vi "8-bit video export-generate images.vi"(0 "AVI2 split file ref":T3, 1 "rgb Image":T2, 2 "Caller (exporter)":enum16{"Viewer", "Exporter"}(ring)=enum."Exporter", 3 "Initial frame":bool, 5 "Gobal frame number in time series data /master video (1 based)":i32, 7 "Split time series file frame index (0 based)":u32, 9 "I16 Image ref in":T2, 11 "Ctrl refs":T1, 12 "U8 Image ref in":T2, 13 "Whole dataset":bool) -> (4 "U8 Image":T2, 6 "Max intensity value":dbl, 10 "I16 Image":T2, 15 "error out":errorcluster)   [LabVIEW 2020]
uses:
  <vilib>/vision/Avi.llb/IMAQ AVI2 Refnum.ctl
  <vilib>/vision/Image Controls.llb/IMAQ Image.ctl
  Typedefs/8-bit video export window ctrl refs.ctl
  Patch-Vol video generator/Typedefs/Bright-Contr-Gamma cluster.ctl
  Typedefs/Speed graph behaviour enum.ctl
panel:
  in  "Output X Resolution per Tier":i32=500
  out "Image Pixels (U32)":u32[][](array[numeric])
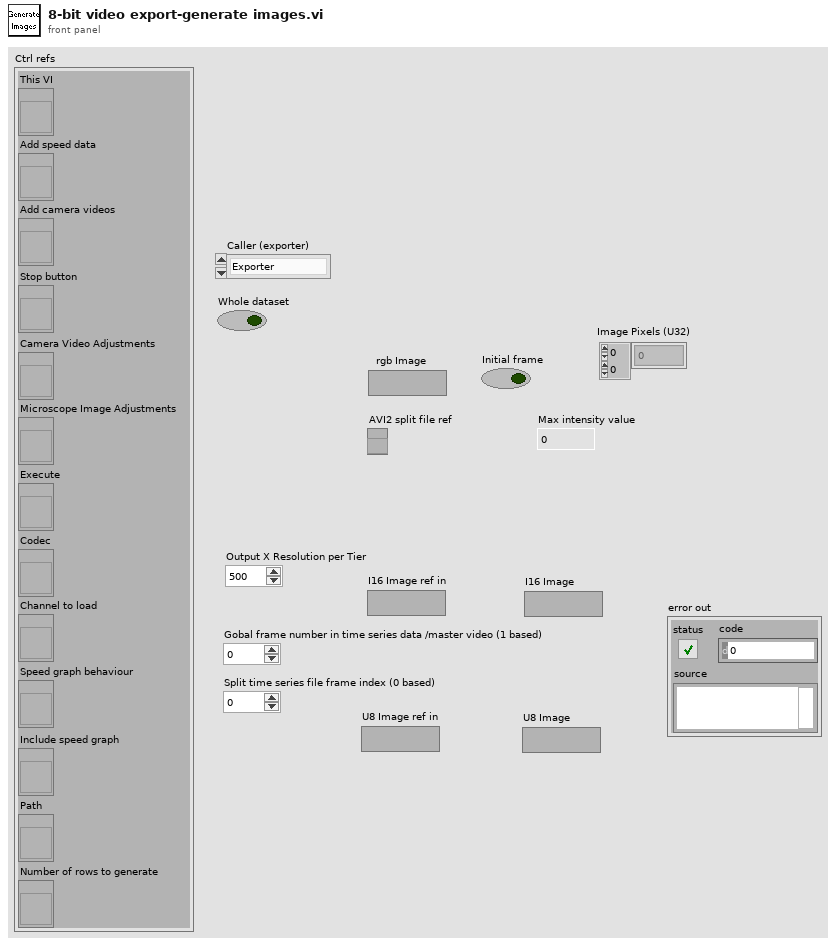
[diagram p1: front panel]
types:
  T1 = typedef "8-bit video export window ctrl refs.ctl" = cluster{"This VI":refnum<vi>, "Add speed data":refnum<vi>, "Add camera videos":refnum<vi>, "Stop button":refnum<vi>, "Camera Video Adjustments":refnum<vi>, "Microscope Image Adjustments":refnum<vi>, "Execute":refnum<vi>, "Codec":refnum<vi>, "Channel to load":refnum<vi>, "Speed graph behaviour":refnum<vi>, "Include speed graph":refnum<vi>, "Number of rows to generate":refnum<vi>, "Path":refnum<vi>}
  T2 = typedef "IMAQ Image.ctl" = refnum<image>
  T3 = typedef "IMAQ AVI2 Refnum.ctl" = refnum<k20>
  T4 = typedef "Bright-Contr-Gamma cluster.ctl" = cluster{"Brightness":sgl, "Contrast":sgl, "Gamma":sgl}
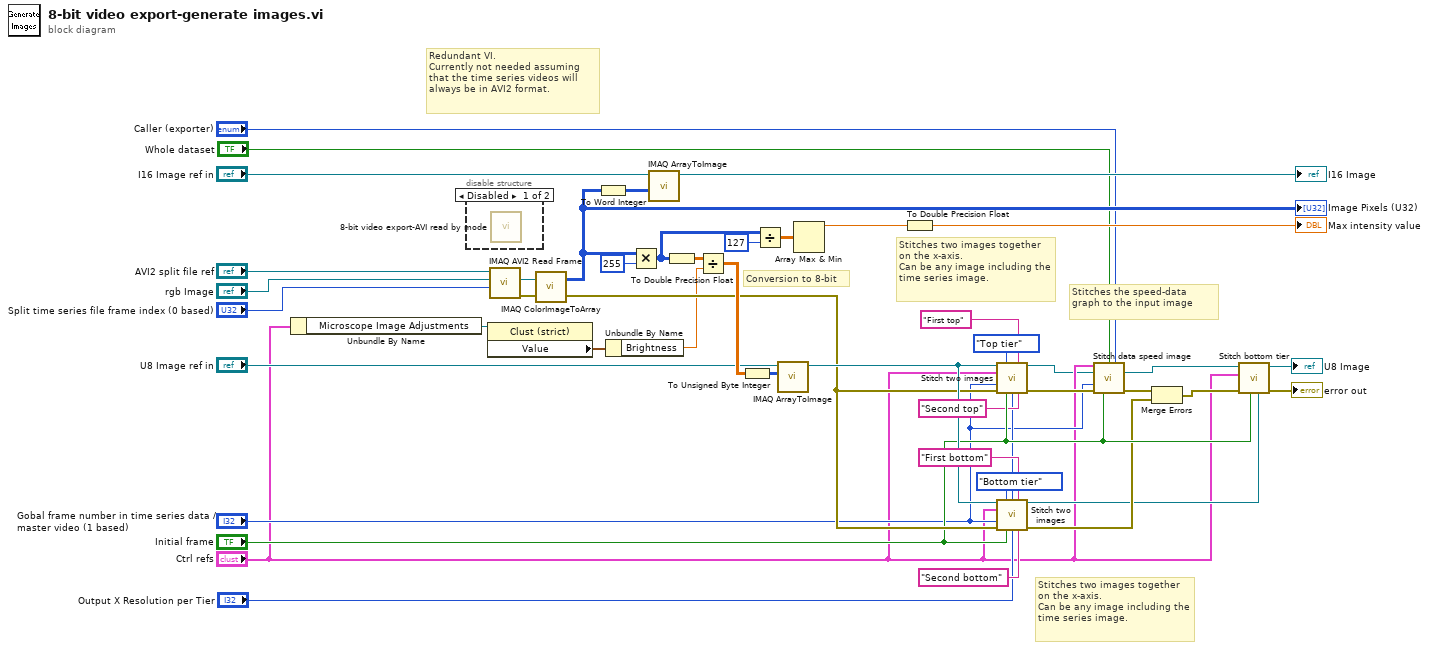
[diagram p0: block diagram]
diagram:
  # "Redundant VI.\nCurrently not needed assuming that the time series videos will always be in AVI2 format."
  # "Stitches two images together on the x-axis.\nCan be any image including the time series image."
  # "Stitches two images together on the x-axis.\nCan be any image including the time series image."
  # "Conversion to 8-bit"
  # "Stitches the speed-data graph to the input image"
  n1 = Unbundle By Name("Ctrl refs") -> ("Microscope Image Adjustments"=w27:refnum<vi>)
  n2 = disable-structure shown="Disabled" {
    frame Disabled {
      n3 = call "8-bit video export-AVI read by mode.vi"() -> ()  [unwired: 9 in, 3 out]
    }
    frame Enabled {
    }
  }
  n4 = property class="Clust (strict)"(reference=w27) -> ("Value"=w4:T4)  [unwired: 1 in, 2 out]
  n5 = call "IMAQ AVI2 Read Frame"("Frame Number"="Split time series file frame index (0 based)", "Image"="rgb Image", "AVI Refnum"="AVI2 split file ref") -> ("error out"=w35:errorcluster, "Image Out"=w36:T2)  [unwired: 6 in, 1 out]
  n6 = call "IMAQ ColorImageToArray"("Image"=w36, "error in (no error)"=w35) -> ("Image Pixels (U32)"=w43:u32[][], "error out"=w22:errorcluster)  [unwired: 1 in, 2 out]
  "Image Pixels (U32)" <- w43
  n7 = To Word Integer(number=w43) -> (16bit integer=w38:i16[][])
  n8 = Unbundle By Name(w4) -> ("Brightness"=w3:sgl)
  n9 = Multiply(x=w43, y=u32 255 ("Number of frames")) -> (x*y=w30:u32[][])
  n10 = call "IMAQ ArrayToImage"("Image Pixels (I16)"=w38, "Image"="I16 Image ref in") -> ("Image Out"=→"I16 Image":T2)  [unwired: 8 in, 1 out]
  n11 = To Double Precision Float(number=w30) -> (double precision float=w41:dbl[][])
  n12 = Divide(x=w41, y=w3) -> (x/y=w44:dbl[][])
  n13 = To Unsigned Byte Integer(number=w44) -> (unsigned 8bit integer=w39:u8[][])
  n14 = Divide(x=w30, y=i8 127 ("Numeric")) -> (x/y=w29:dbl[][])
  n15 = call "IMAQ ArrayToImage"("Image Pixels (U8)"=w39, "Image"="U8 Image ref in") -> ("Image Out"=w25:T2)  [unwired: 8 in, 1 out]
  n16 = Array Max & Min(array=w29) -> (max value=w32:dbl)  [unwired: 3 out]
  n17 = To Double Precision Float(number=w32) -> (double precision float=→"Max intensity value":dbl)
  n18 = call "Stitch two images.vi"("Timelapse Image in"=w25, "Which tier?"=enum16{"Top tier", "Bottom tier"}."Top tier", "Name for resampled Image 1"="First top" ("Resampled Image Name"), "Ctrl refs"="Ctrl refs", "Gobal frame number in Timelapse data/master video (1 based)"="Gobal frame number in time series data /master video (1 based)", "error in (no error)"=w22, "Initial frame"="Initial frame", "Output X Resolution"="Output X Resolution per Tier", "Name for resampled Image 2"="Second top" ("Resampled Image Name 2")) -> ("Bottom tier Stitched Image"=w6:T2, "error out"=w26:errorcluster)  [unwired: 5 in]
  n19 = call "Stitch two images.vi"("Timelapse Image in"=w25, "Which tier?"=enum16{"Top tier", "Bottom tier"}."Bottom tier", "Name for resampled Image 1"="First bottom" ("Resampled Image Name"), "Ctrl refs"="Ctrl refs", "Gobal frame number in Timelapse data/master video (1 based)"="Gobal frame number in time series data /master video (1 based)", "error in (no error)"=w22, "Initial frame"="Initial frame", "Output X Resolution"="Output X Resolution per Tier", "Name for resampled Image 2"="Second bottom" ("Resampled Image Name 2")) -> ("Bottom tier Stitched Image"=w15:T2, "error out"=w17:errorcluster)  [unwired: 5 in]
  n20 = call "Stitch data speed image.vi"("Ctrl refs"="Ctrl refs", "Whole dataset"="Whole dataset", "Caller"="Caller (exporter)", "Microscope image"=w6, "Global frame number in master video(s)"="Gobal frame number in time series data /master video (1 based)", "error in (no error)"=w26, "Initial frame"="Initial frame") -> ("Stitched Image"=w5:T2, "error out"=w18:errorcluster)  [unwired: 7 in]
  n21 = Merge Errors(w18, w17) -> (w16:errorcluster)
  n22 = call "Stitch bottom tier.vi"("Bottom tier Stitched Image"=w15, "Initial frame"="Initial frame", "error in (no error)"=w16, "Ctrl refs"="Ctrl refs", "Input stitched image"=w5) -> ("error out"=→"error out":errorcluster, "Stitched Image"=→"U8 Image":T2)  [unwired: 5 in]
